vi "solar_addon Launch.vi"(8 "error in (no error)":errorcluster, 9 "SOLAR Refnum":T1, 11 "Menu Label":string) -> (0 "error out":errorcluster, 1 "Exists?":bool, 3 "Addons (vi,title)":string[][](array[string]))   [LabVIEW 2018]
doc: "This launches a SOLAR addon by menu label (i.e. Tools > Menu Title) If the Addon is not found, this does nothing."
uses:
  solar/solar_ctl SOLAR Refnum.ctl
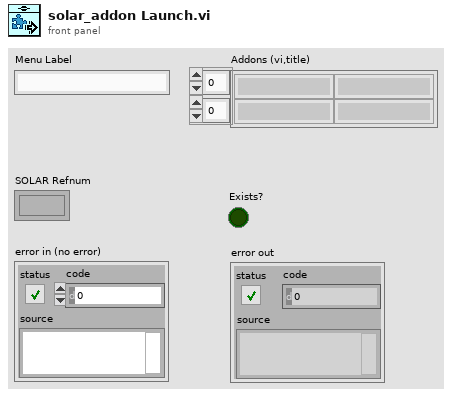
[diagram p1: front panel]
types:
  T1 = typedef "solar_ctl SOLAR Refnum.ctl" = refnum<k1>
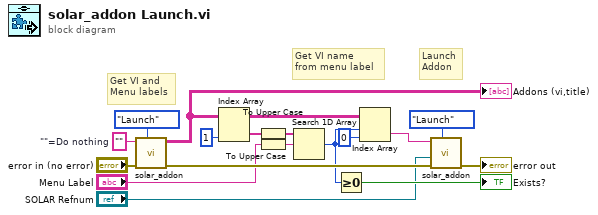
[diagram p0: block diagram]
diagram:
  w16 = ""  # ""=Do nothing
  # "Launch\nAddon"
  # "Get VI name\nfrom menu label"
  # "Get VI and \nMenu labels"
  n1 = call "solar_addon.vi"("Action (Launch)"=enum8{"Launch", "Initialize", "Shutdown"}."Launch", "error in (no error)"="error in (no error)", "Launch Addon VI"=w16) -> ("error out"=w13:errorcluster, "Addons (vi,title)"=w4:string[][])  [unwired: 7 in]
  "Addons (vi,title)" <- w4
  n2 = Index Array(array=w4, index (col)=1 ("disabled index (col)")) -> (element=w10:string[])  [unwired: 1 in]
  n3 = To Upper Case(1:w10) -> (0:w8:string[])
  n4 = To Upper Case(1:"Menu Label") -> (0:w7:string)
  n5 = Search 1D Array(1D array=w8, element=w7) -> (index of element=w3:i32)  [unwired: 1 in]
  n6 = Greater Or Equal To 0?(x=w3) -> (x >= 0?=→"Exists?":bool)
  n7 = Index Array(array=w4, index (row)=w3, index (col)=0 ("disabled index (col)")) -> (element=w5:string)
  n8 = call "solar_addon.vi"("Action (Launch)"=enum8{"Launch", "Initialize", "Shutdown"}."Launch", "error in (no error)"=w13, "SOLAR Refnum"="SOLAR Refnum", "Launch Addon VI"=w5) -> ("error out"=→"error out":errorcluster)  [unwired: 6 in, 1 out]
